vi "Digital Output.vi"(8 "error in":errorcluster, 11 "DAQmx OutPut Setting":T1) -> (0 "error out":errorcluster, 1 "Exit":bool)   [LabVIEW 2015]
uses:
  <vilib>/DAQmx/write.llb/DAQmx Write (Digital 2D Bool NChan 1Samp NLine).vi
  <vilib>/DAQmx/write.llb/DAQmx Write (Digital 1D Bool 1Chan 1Samp).vi
  <vilib>/DAQmx/create/channels.llb/DAQmx Create Channel (DO-Digital Output).vi
  Galobal variable_TI.vi
  <vilib>/DAQmx/miscellaneous.llb/DAQmx Fill In Error Info.vi
panel:
  out "error out 2":errorcluster
  out "array":tag[](array[tag])
  out "*(type *) &x":tag
  out "Digital Output":bool[](array[boolean])
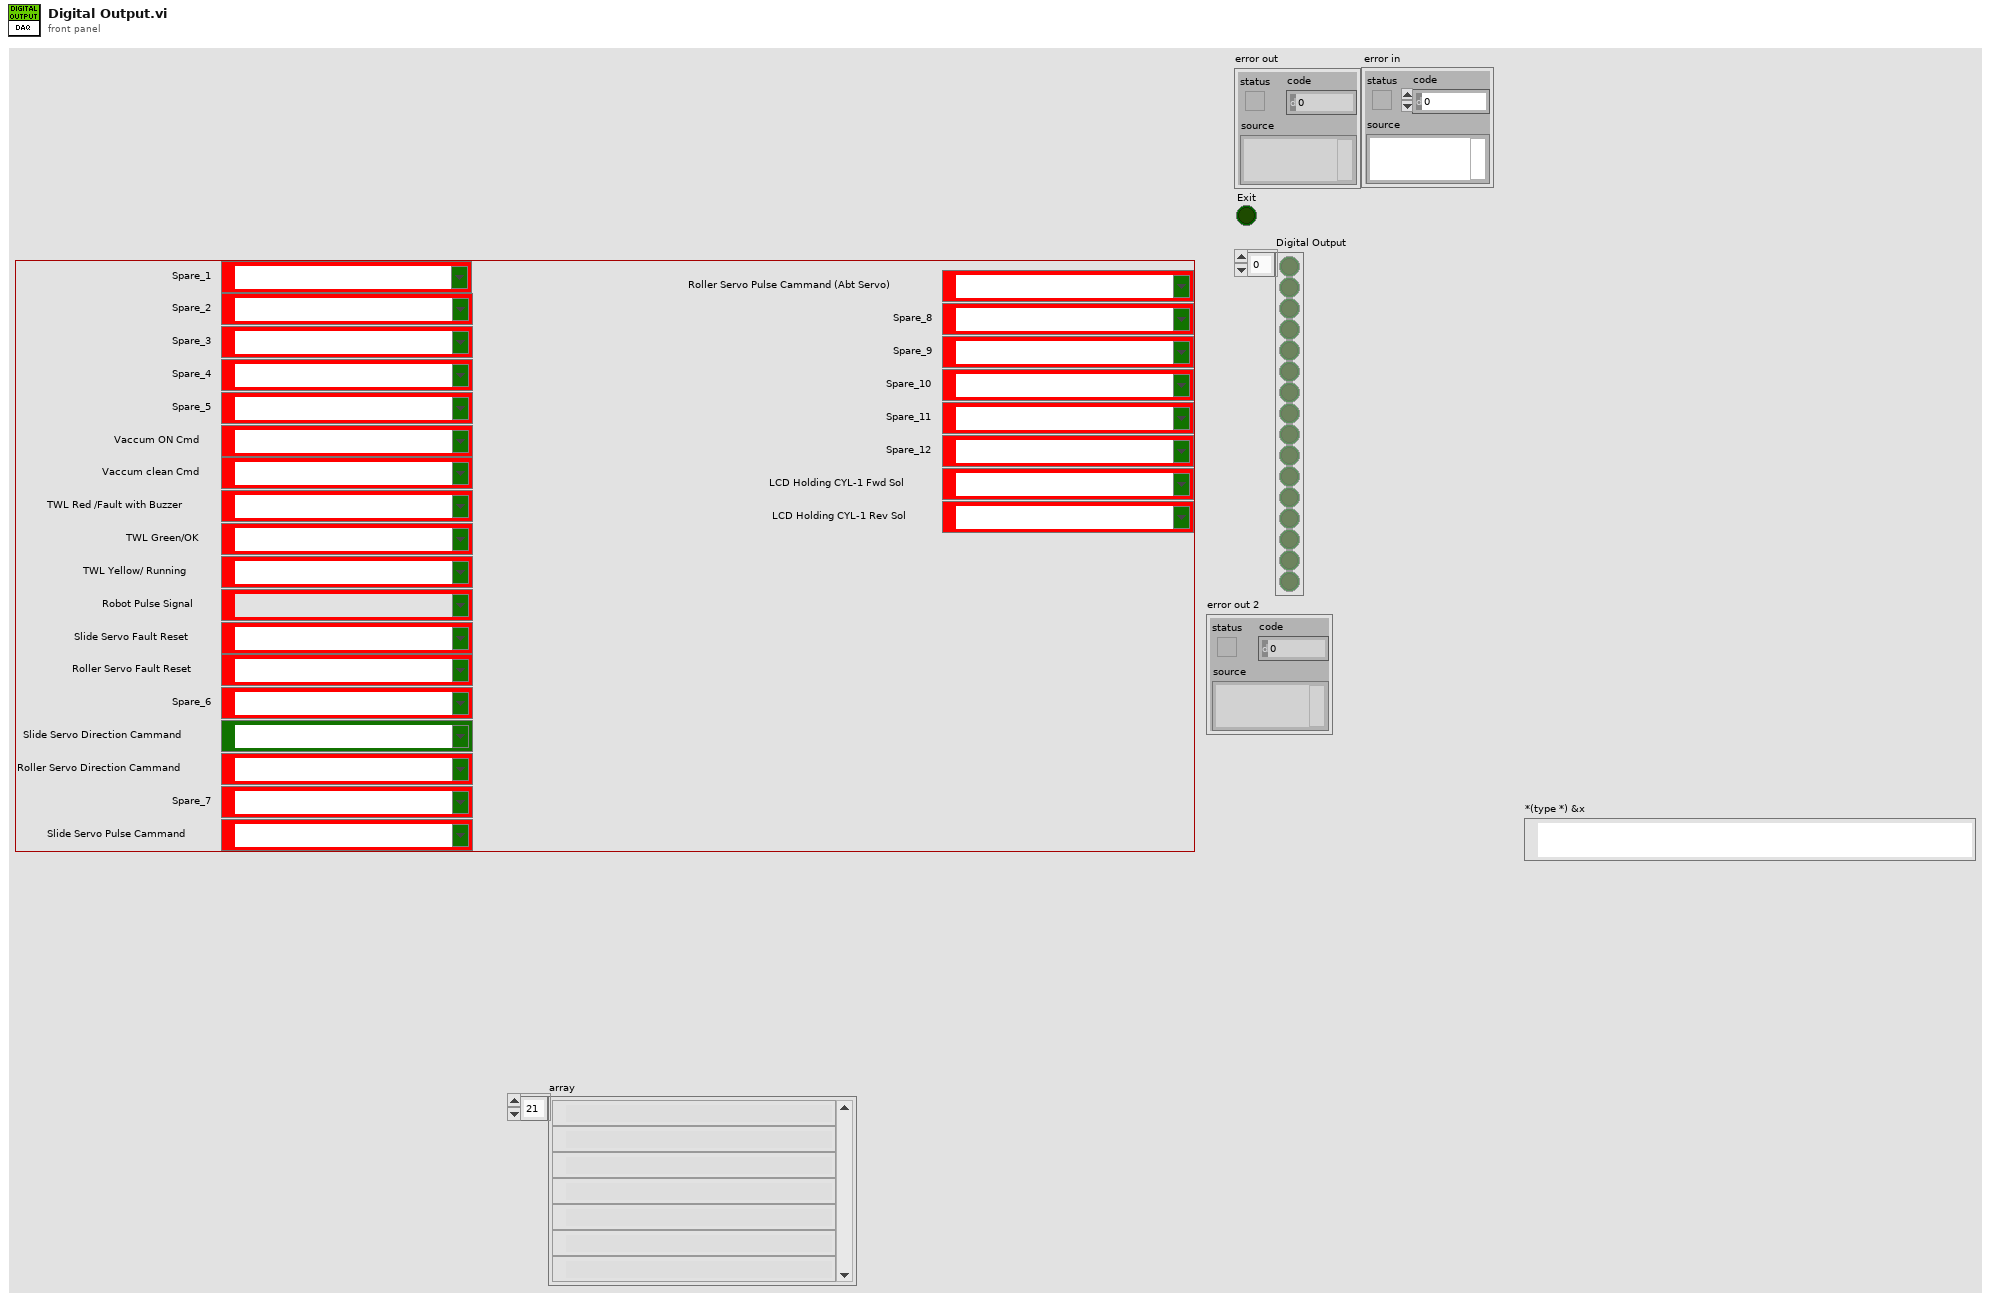
[diagram p1: front panel]
types:
  T1 = cluster{"DAQmx OutPut_00":tag, "DAQmx OutPut_01":tag, "DAQmx OutPut_02":tag, "DAQmx OutPut_03":tag, "DAQmx OutPut_04":tag, "DAQmx OutPut_05":tag, "DAQmx OutPut_06":tag, "DAQmx OutPut_07":tag, "DAQmx OutPut_08":tag, "DAQmx OutPut_09":tag, "DAQmx OutPut_10":tag, "DAQmx OutPut_11":tag, "DAQmx OutPut_12":tag, "DAQmx OutPut_13":tag, "DAQmx OutPut_14":tag, "DAQmx OutPut_15":tag, "DAQmx OutPut_16":tag, "DAQmx OutPut_17":tag, "DAQmx OutPut_18":tag, "DAQmx OutPut_19":tag, "DAQmx OutPut_20":tag, "DAQmx OutPut_21":tag, "DAQmx OutPut_22":tag, "DAQmx OutPut_23":tag, "DAQmx OutPut_12 2":tag, "DAQmx OutPut_13 2":tag}
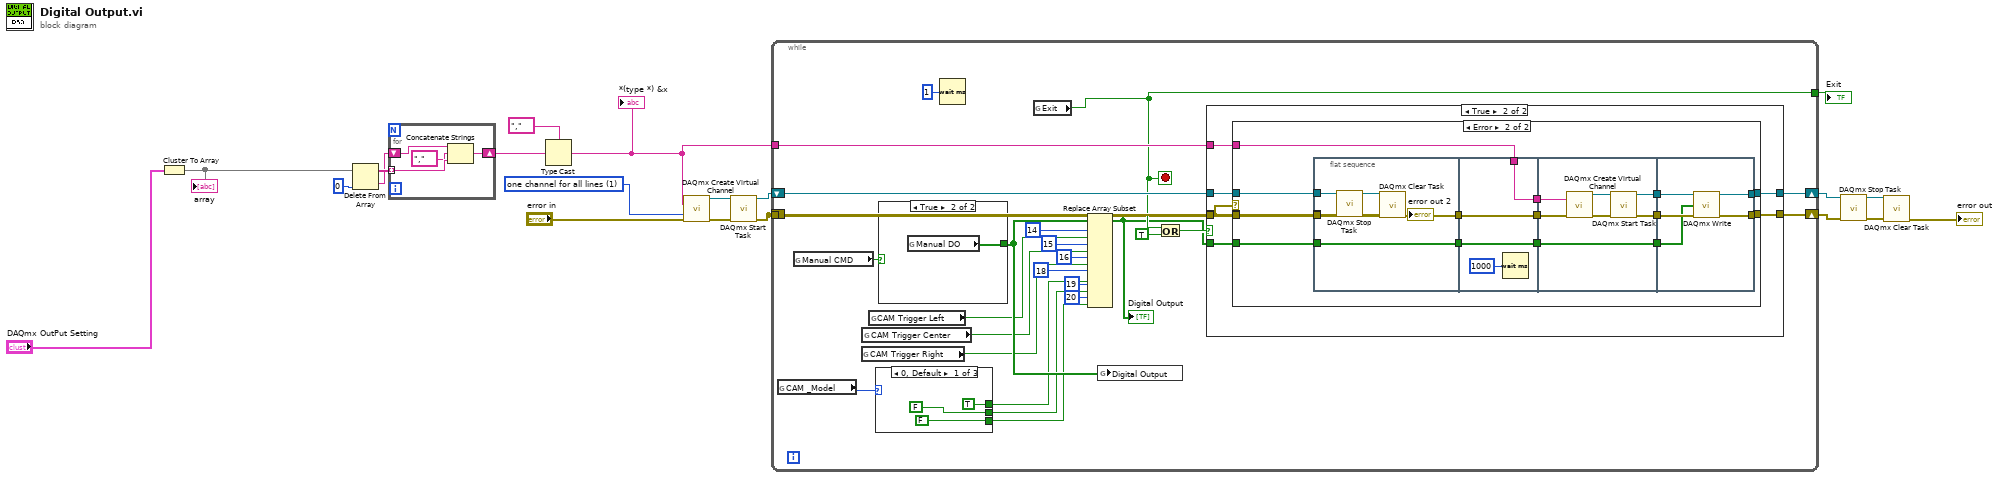
[diagram p0: block diagram]
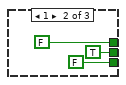
[diagram p2: hidden frame]
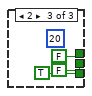
[diagram p3: hidden frame]
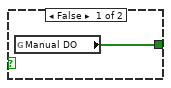
[diagram p4: hidden frame]
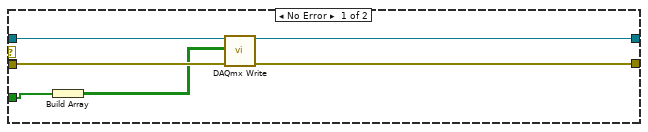
[diagram p6: hidden frame]
diagram:
  w5 = 1 items=["one channel for each line", "one channel for all lines"] ("line grouping")
  n1 = Cluster To Array(cluster="DAQmx OutPut Setting") -> (array=w3:tag[])
  "array" <- w3
  n2 = Delete From Array(array=w3, index=0) -> (deleted portion=w8:tag, array with subset deleted=w10:tag[])  [unwired: 1 in]
  n3 = for {
    tunnel: w10 -> [w23] mode=indexing
    shift-right: [w21] -> w6
    shift-left: w8 -> [w24]
    n4 = Concatenate Strings(w24, tag "," ("1."), w23) -> (w21:string)
  }
  n5 = Type Cast(type=tag "," ("1."), x=w6) -> (*(type *) &x=w4:tag)
  "*(type *) &x" <- w4
  n6 = call-poly <vilib>:"DAQmx Create Virtual Channel.vi"("lines"=w4, "line grouping"=w5, "error in"="error in") -> ("task out"=w20:refnum<k21>, "error out"=w19:errorcluster)  [unwired: 2 in, 9 out]
  n7 = call <vilib>:"DAQmx Start Task.vi"("task/channels in"=w20, "error in"=w19) -> ("task out"=w16:refnum<k21>, "error out"=w1:errorcluster)  [unwired: 12 out]
  n8 = while {
    shift-right: [w48] -> w14
    shift-left: w1 -> [w47]
    shift-right: [w49] -> w15
    shift-left: w16 -> [w50]
    tunnel: w4 -> [w46]
    tunnel: [w43] -> w11
    tunnel: w1 -> [w25]
    stop <- w43 stop-if-true
    n9 = global read "Galobal variable_TI.vi" "CAM _Model"() -> (w38:i32)
    n10 = global read "Galobal variable_TI.vi" "Manual CMD"() -> (w42:bool)
    n11 = global read "Galobal variable_TI.vi" "CAM Trigger Right"() -> (w26:bool)
    n12 = global read "Galobal variable_TI.vi" "CAM Trigger Center"() -> (w27:bool)
    n13 = global read "Galobal variable_TI.vi" "CAM Trigger Left"() -> (w28:bool)
    n14 = case shown="0, Default" w38 {
      tunnel: [TRUE FALSE FALSE] -> w32
      tunnel: [FALSE TRUE FALSE] -> w34
      tunnel: [FALSE FALSE TRUE] -> w33
      frame 0, Default {
      }
      frame 1 {
      }
      frame 2 {
        (unwired) 20 ("index")
      }
    }
    n15 = case shown="True" w42 {
      tunnel: [w60 w61] -> w40
      frame False {
        n16 = global read "Galobal variable_TI.vi" "Manual DO"() -> (w60:bool[])
      }
      frame True {
        n17 = global read "Galobal variable_TI.vi" "Manual DO"() -> (w61:bool[])
      }
    }
    n18 = Wait (ms)(milliseconds to wait=u32 1) -> ()  [unwired: 1 out]
    n19 = global read "Galobal variable_TI.vi" "Exit"() -> (w43:bool)
    n20 = Replace Array Subset(array=w40, new element #1=w28, index #1=14 ("index"), new element #2=w27, index #2=15 ("index"), new element #3=w26, index #3=16 ("index"), new element #4=w32, index #4=18 ("index"), new element #5=w34, index #5=19 ("index"), new element #6=w33, index #6=20 ("index")) -> (w39:bool[])
    "Digital Output" <- w39
    n21 = global write "Galobal variable_TI.vi" "Digital Output"(w40) -> ()
    n22 = Or(x=w43, y=TRUE) -> (x .or. y?=w45:bool)
    n23 = case shown="True" w45 {
      tunnel: w50 -> [w63 w70]
      tunnel: [w63 w69] -> w49
      tunnel: [w62 w68] -> w48
      tunnel: w47 -> [w62 w67]
      tunnel: w46 -> [_ w66]
      tunnel: w39 -> [_ w65]
      tunnel: w25 -> [_ w64]
      frame False {
      }
      frame True {
        n24 = case shown="Error" w67 {
          tunnel: w70 -> [w76 w91]
          tunnel: w67 -> [w75 w90]
          tunnel: [w74 w88] -> w69
          tunnel: [w73 w89] -> w68
          tunnel: w66 -> [_ w85]
          tunnel: w65 -> [w72 w82]
          tunnel: w64 -> [_ w77]
          frame No Error {
            n25 = Build Array(w72) -> (w71:bool[][])
            n26 = call-poly <vilib>:"DAQmx Write.vi"("task/channels in"=w76, "data"=w71, "error in"=w75) -> ("task out"=w74:refnum<k21>, "error out"=w73:errorcluster)  [unwired: 1 in, 10 out]
          }
          frame Error {
            n27 = flat-sequence {
              tunnel: w91 -> [w96]
              tunnel: w90 -> [w95]
              tunnel: w82 -> [w94]
              tunnel: [w94] -> w81
              tunnel: [w92] -> w78
              tunnel: w77 -> [w92]
              tunnel: [w99] -> w87
              tunnel: [w101] -> w86
              tunnel: w85 -> [w101]
              tunnel: w81 -> [w100]
              tunnel: [w100] -> w80
              tunnel: w78 -> [w99]
              tunnel: w87 -> [w105]
              tunnel: w86 -> [w104]
              tunnel: [w107] -> w84
              tunnel: [w106] -> w83
              tunnel: w80 -> [w103]
              tunnel: [w103] -> w79
              tunnel: [w112] -> w88
              tunnel: [w113] -> w89
              tunnel: w84 -> [w114]
              tunnel: w83 -> [w111]
              tunnel: w79 -> [w110]
              frame #0 {
                n28 = call <vilib>:"DAQmx Stop Task.vi"("task/channels in"=w96, "error in"=w95) -> ("task out"=w97:refnum<k21>, "error out"=w98:errorcluster)  [unwired: 12 out]
                n29 = call <vilib>:"DAQmx Clear Task.vi"("task in"=w97, "error in"=w98) -> ("error out"=→"error out 2":errorcluster)  [unwired: 13 out]
              }
              frame #1 {
                n30 = Wait (ms)(milliseconds to wait=u32 1000) -> ()  [unwired: 1 out]
              }
              frame #2 {
                n31 = call-poly <vilib>:"DAQmx Create Virtual Channel.vi"("lines"=w104, "error in"=w105) -> ("task out"=w109:refnum<k21>, "error out"=w108:errorcluster)  [unwired: 3 in, 9 out]
                n32 = call <vilib>:"DAQmx Start Task.vi"("task/channels in"=w109, "error in"=w108) -> ("task out"=w106:refnum<k21>, "error out"=w107:errorcluster)  [unwired: 12 out]
              }
              frame #3 {
                n33 = call-poly <vilib>:"DAQmx Write.vi"("task/channels in"=w111, "data"=w110, "error in"=w114) -> ("task out"=w112:refnum<k21>, "error out"=w113:errorcluster)  [unwired: 1 in, 10 out]
              }
            }
          }
        }
      }
    }
  }
  "Exit" <- w11
  n34 = call <vilib>:"DAQmx Stop Task.vi"("task/channels in"=w15, "error in"=w14) -> ("task out"=w18:refnum<k21>, "error out"=w17:errorcluster)  [unwired: 12 out]
  n35 = call <vilib>:"DAQmx Clear Task.vi"("task in"=w18, "error in"=w17) -> ("error out"=→"error out":errorcluster)  [unwired: 13 out]
